vi "Set Minimum Voltage.vi"(8 "error in (no error)":errorcluster, 10 "voltage (5V)":u16=5000, 11 "DC Brick in":refnum<class "DC Brick.lvclass">) -> (0 "error out":errorcluster, 3 "DC Brick out":refnum<class "DC Brick.lvclass">)   [LabVIEW 2011, in "Tinkerforge.lvlib" / "DC Brick.lvclass"]
doc: "This VI sets the minimum voltage in mV, below which the CALLBACK_UNDER_VOLTAGE callback is triggered. The minimum possible value that works with the DC Brick is 5V. You can use this function to detect the discharge of a battery that is used to drive the motor. If you have a fixed power supply, you likely do not need this functionality.\n\nThe default value is 5V."
uses:
  DC Brick.lvclass
  Device/Device.lvclass
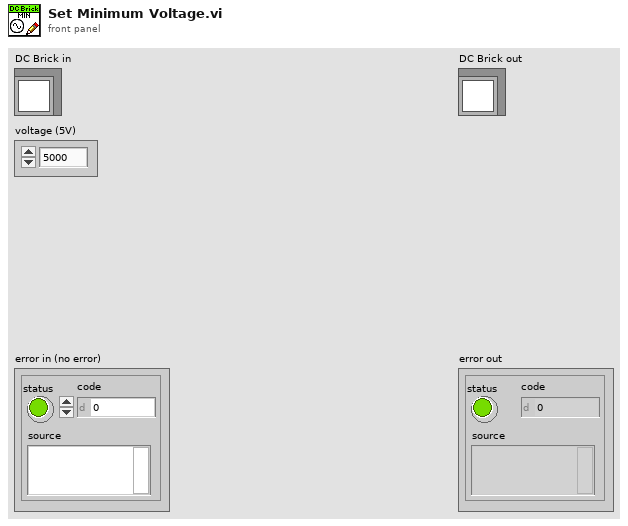
[diagram p1: front panel]
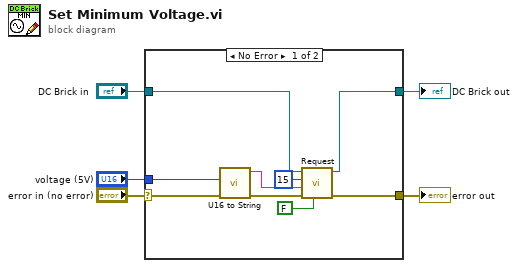
[diagram p0: block diagram]
diagram:
  n1 = case shown="No Error" "error in (no error)" {
    selector: "error in (no error)" -> [w9 w16]
    tunnel: [w10 w16] -> w4
    tunnel: [w13 w15] -> w2
    tunnel: "DC Brick in" -> [w14 w15]
    tunnel: "voltage (5V)" -> [w8 _]
    frame No Error {
      n2 = call "U16 to String.vi"("Error In"=w9, "U16"=w8) -> ("Error Out"=w7:errorcluster, "String out"=w6:string)  [unwired: 8 in]
      n3 = call "Request.vi"("Response"=FALSE, "error in (no error)"=w7, "Data"=w6, "Function ID"=u8 15, "Device in"=w14) -> ("error out"=w10:errorcluster, "Device out"=w13:refnum<class "DC Brick.lvclass">)  [unwired: 2 in, 3 out]
    }
    frame Error {
    }
  }
  "error out" <- w4
  "DC Brick out" <- w2
